vi "offset shift.vi"(7 "read writ":string(combo), 8 "na/V":dbl=500.0, 9 "na/V 2":dbl=1000.0, 10 "field change wait(s)":u32=5, 11 "charge state":dbl=3.0) -> (0 "field change wait(s) out":u32, 1 "na/V 2out":dbl, 2 "na/V out":dbl, 3 "charge state out":dbl)   [LabVIEW 2016]
doc: "allows values to be reset after reload of stable current"
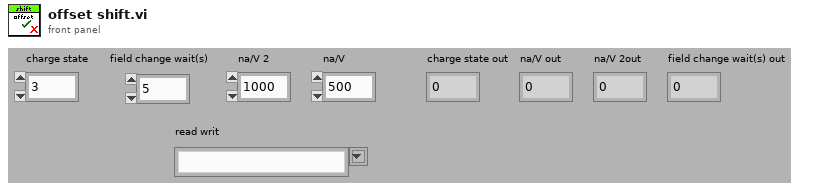
[diagram p1: front panel]
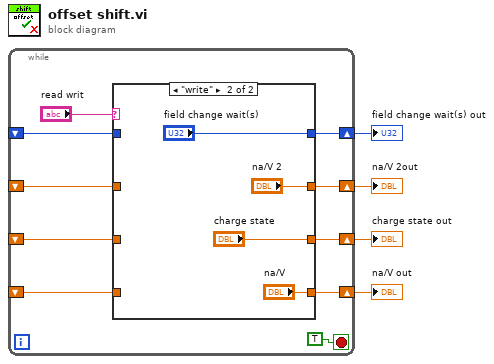
[diagram p0: block diagram]
diagram:
  n1 = while {
    shift-right: [w12] -> w2
    shift-left: _ -> [w9]
    shift-right: [w13] -> w3
    shift-left: _ -> [w8]
    shift-right: [w14] -> w4
    shift-left: _ -> [w7]
    shift-right: [w11] -> w1
    shift-left: _ -> [w6]
    stop <- TRUE ("stop") stop-if-true
    n2 = case shown="\"write\"" "read writ" {
      tunnel: [w16 "na/V 2"] -> w14
      tunnel: [w17 "na/V"] -> w13
      tunnel: [w18 "charge state"] -> w12
      tunnel: [w15 "field change wait(s)"] -> w11
      tunnel: w9 -> [w18 _]
      tunnel: w8 -> [w17 _]
      tunnel: w7 -> [w16 _]
      tunnel: w6 -> [w15 _]
      frame "read", Default {
      }
      frame "write" {
      }
    }
  }
  "na/V 2out" <- w4
  "na/V out" <- w3
  "charge state out" <- w2
  "field change wait(s) out" <- w1
